vi "TANGO_Example_LV2011.vi"() -> ()   [LabVIEW 2018, in "TangoOWN.lvlib"]
uses:
  SubVIs/AxisControl.ctl
  SubVIs/Axis_Switch.ctl
  TangoOWN.lvlib
  SDK/Tango.lvlib
panel:
  out "CloseWindow":bool
  out "Limit Switches":T1[](array[typedef])
  in  "Calibrate":bool
  in  "RMeasure":bool
  in  "Center":bool
  in  "Tab_Control":enum32{"Control", "Low level"}(tab)
  in  "Analog Output2":i32(slide) scale=0.0..100.0
  in  "Analog Output1":i32(slide) scale=0.0..100.0
  in  "Move absolute":bool
  in  "Destination [mm]":dbl[](array[numeric]) format="%_6g"
  in  "Manual Control":T2[](array[typedef])
  in  "Step Width [mm]":dbl=1.0 min=0.0 format="%_6f"
  in  "Send":bool
  in  "Limits":bool
  out "Return Message":string
  in  "Command":string caption="Send Command"
  in  "Sequence":bool
  in  "Maeander":bool
  in  "Set Zero":bool
  in  "Velocity":bool
  out "MinRange":dbl[](array[numeric])
  out "MaxRange":dbl[](array[numeric])
  out "RMResult":dbl[](array[numeric])
  out "Position":dbl[](array[numeric]) format="%_6f"
  out "Number of Axis":u8=3
  in  "ShProt?":bool=TRUE caption="Show Protocol?"
  in  "Disconnect":bool
  out "Connected?":bool
  in  "Connect":bool
  in  "Baudrate":i32=57600
  in  "VISA-Ressourcename":refnum<visa-resource-name>
  out "Func-Return":i32
  in  "Stopp":bool
  out "error out":errorcluster
  out "State":string="Idle"
  in  "Fehler (Eingang, kein Fehler)":errorcluster
  # "TANGO Example v0.1"
  # "E0"
  # "EE"
  # "X"
  # "Y"
  # "Z"
  # "A"
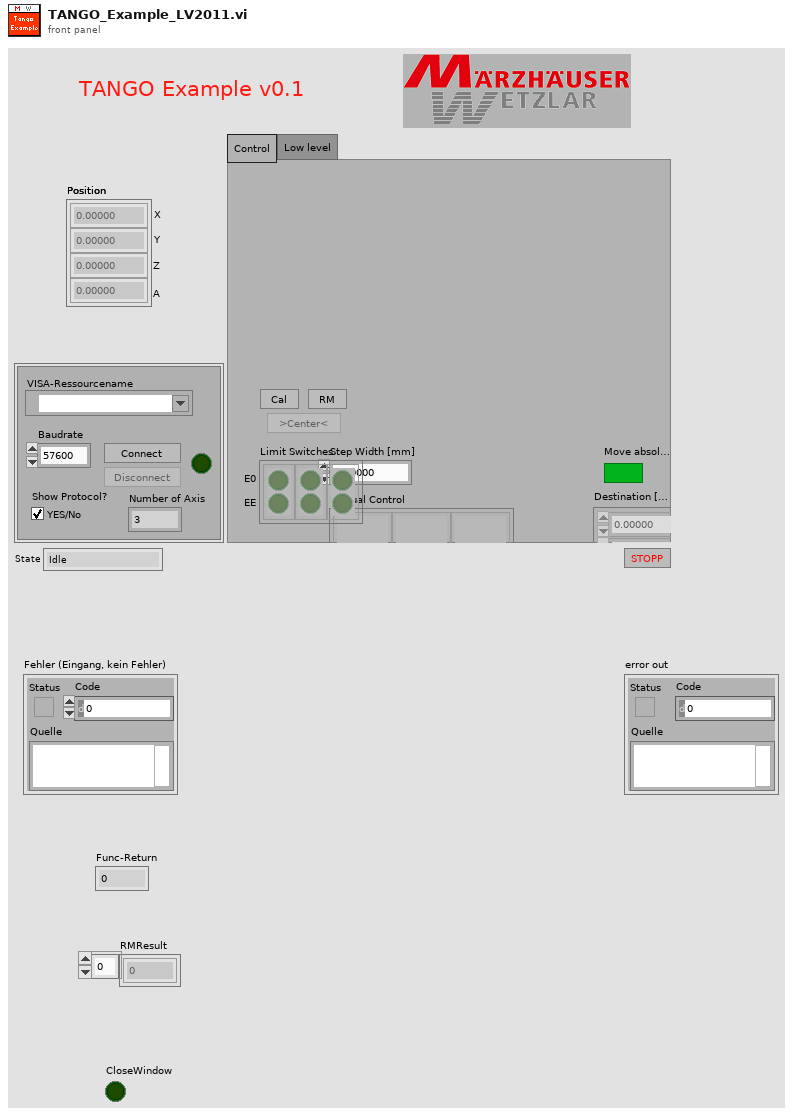
[diagram p1: front panel]
types:
  T1 = typedef "TangoOWN.lvlib/Axis_Switch.ctl" = cluster{"E0":bool, "EE":bool}
  T2 = typedef "TangoOWN.lvlib/AxisControl.ctl" = cluster{"Plus":bool, "Minus":bool}
  T3 = enum8{"Enabled", "Disabled", "Disabled and Grayed Out"}
  T4 = typedef "TangoOWN.lvlib/Maeander_Param.ctl" = cluster{"Number":i32, "X Start":dbl, "Y Start":dbl, "X Size":dbl, "Y Size":dbl}
  T5 = typedef "TangoOWN.lvlib/SequenceParam.ctl" = cluster{"Number of cycles":i32, "Start position":dbl[], "End position":dbl[]}
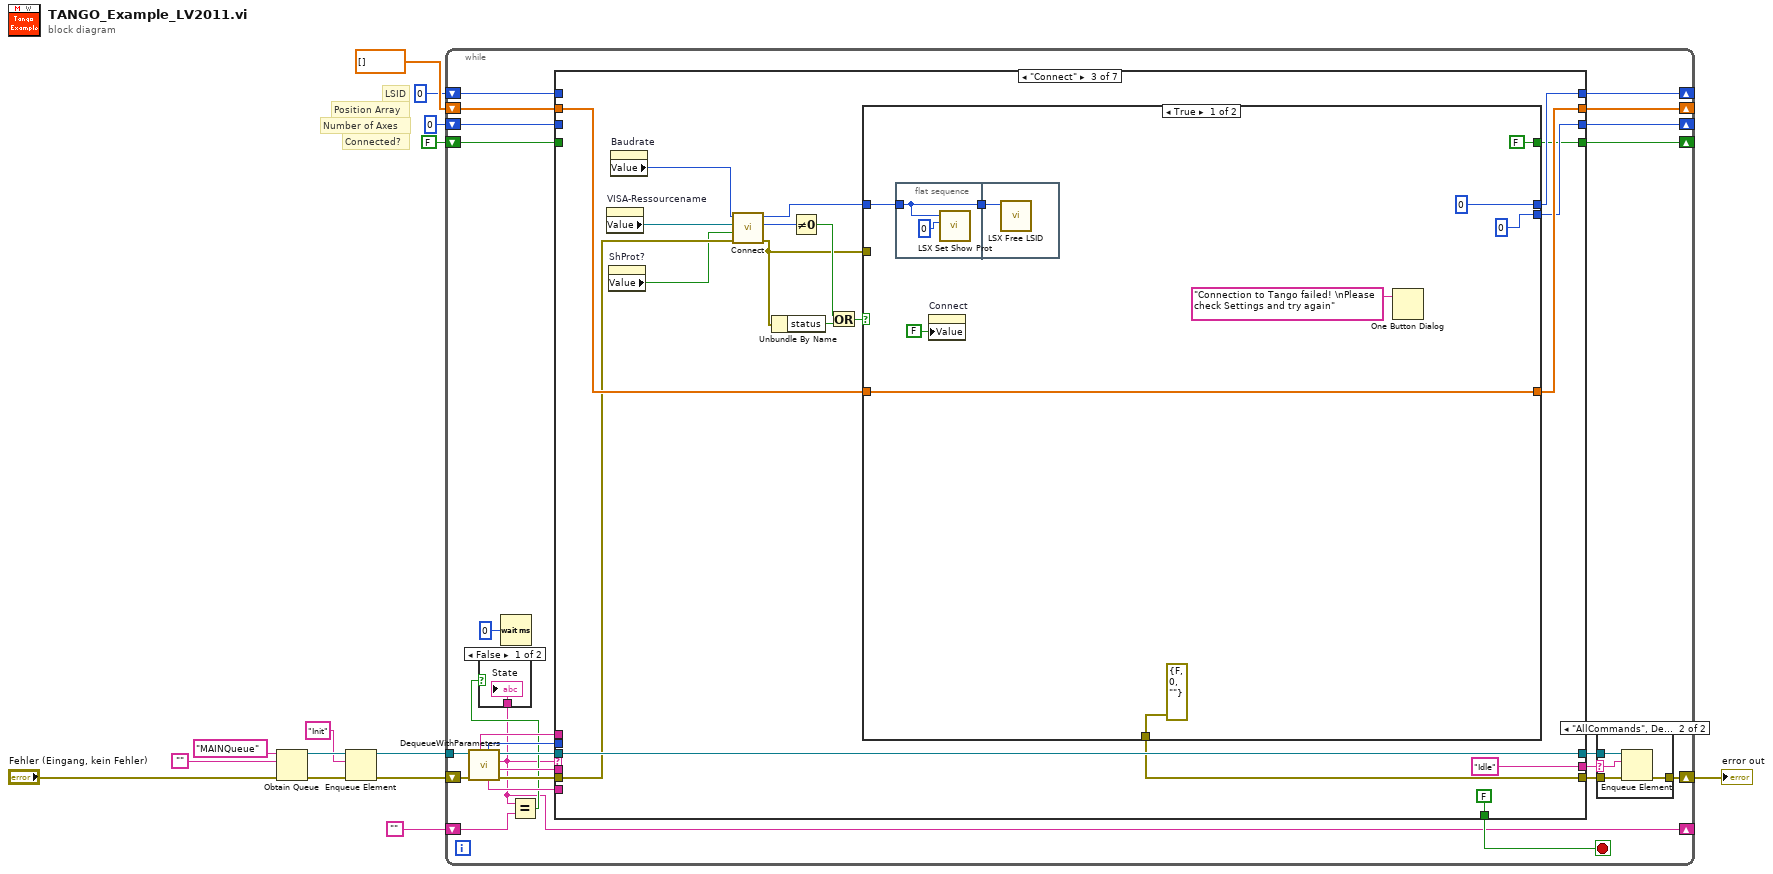
[diagram p0: block diagram]
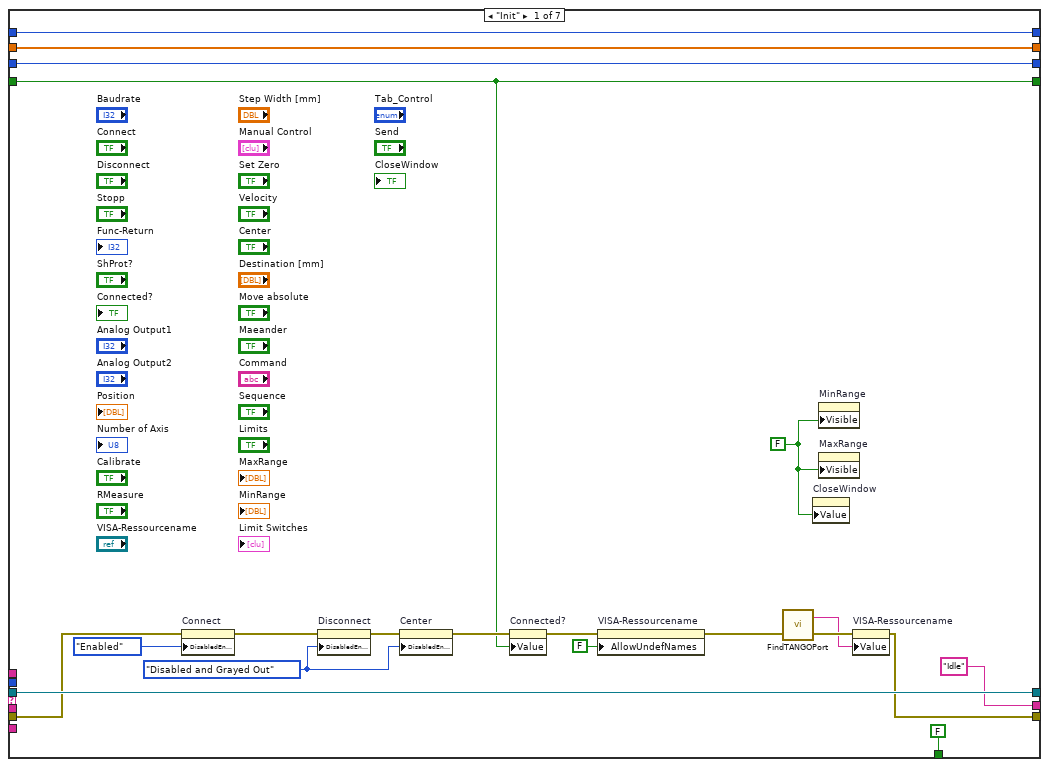
[diagram p4: hidden frame]
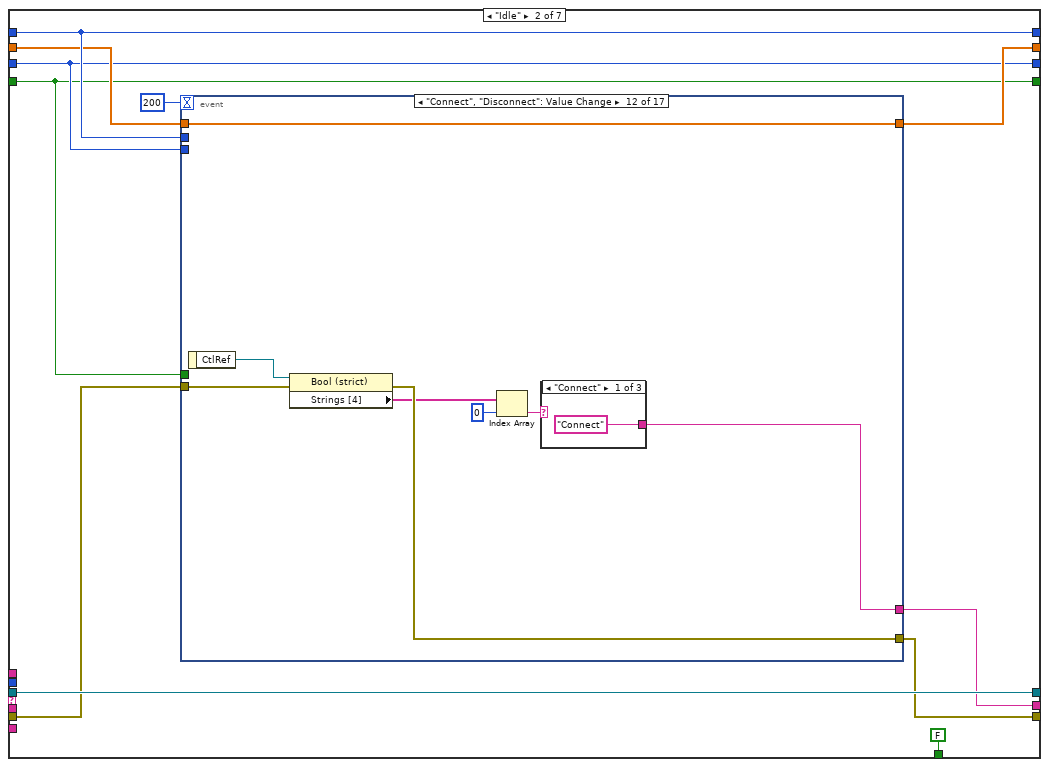
[diagram p5: hidden frame]
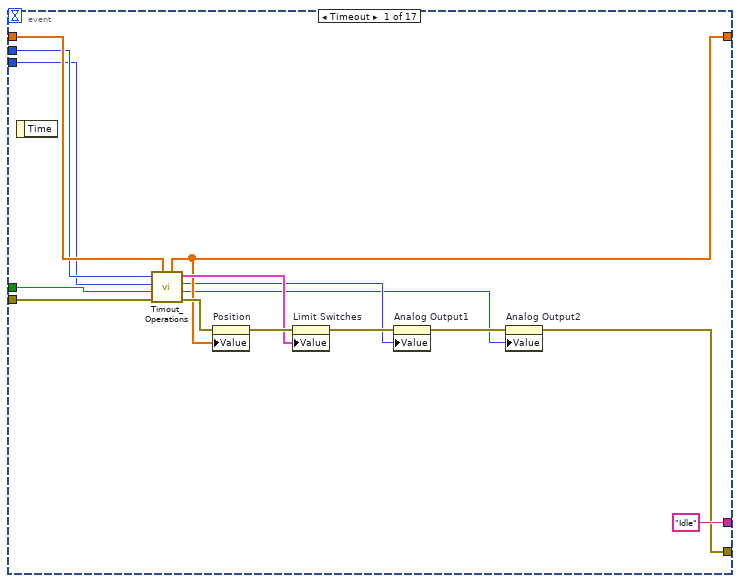
[diagram p6: hidden frame]
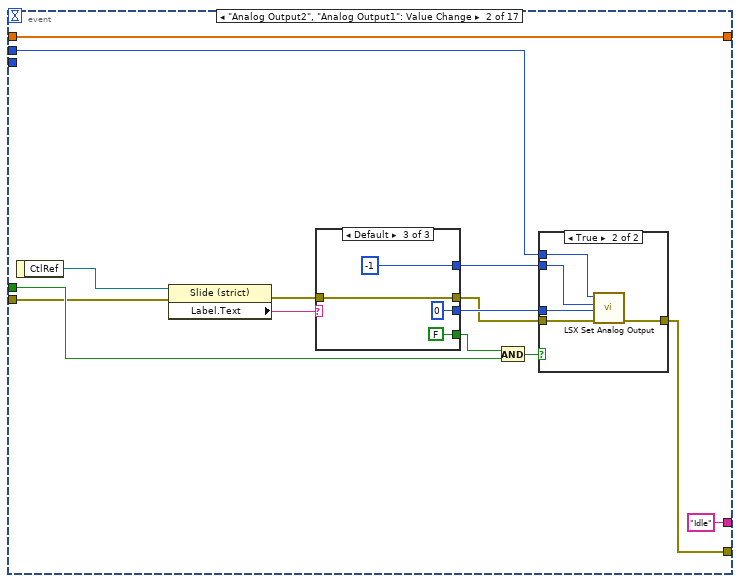
[diagram p7: hidden frame]
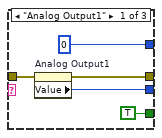
[diagram p8: hidden frame]
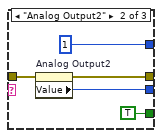
[diagram p9: hidden frame]
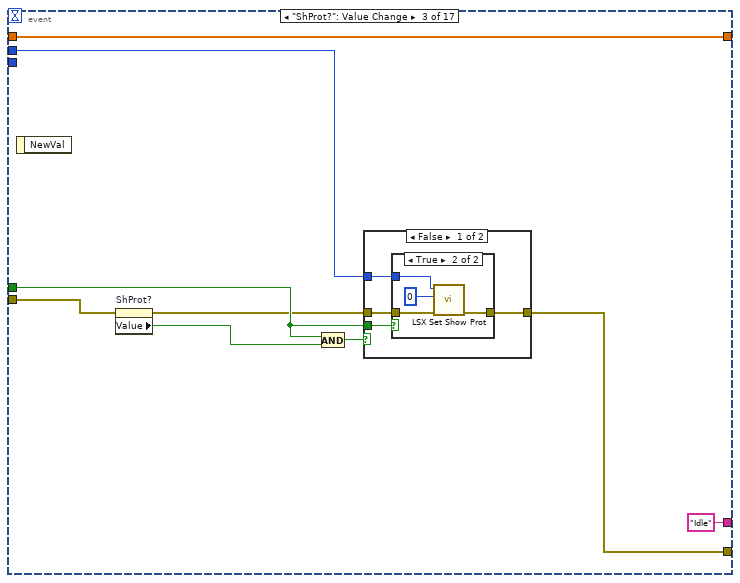
[diagram p11: hidden frame]
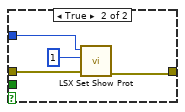
[diagram p13: hidden frame]
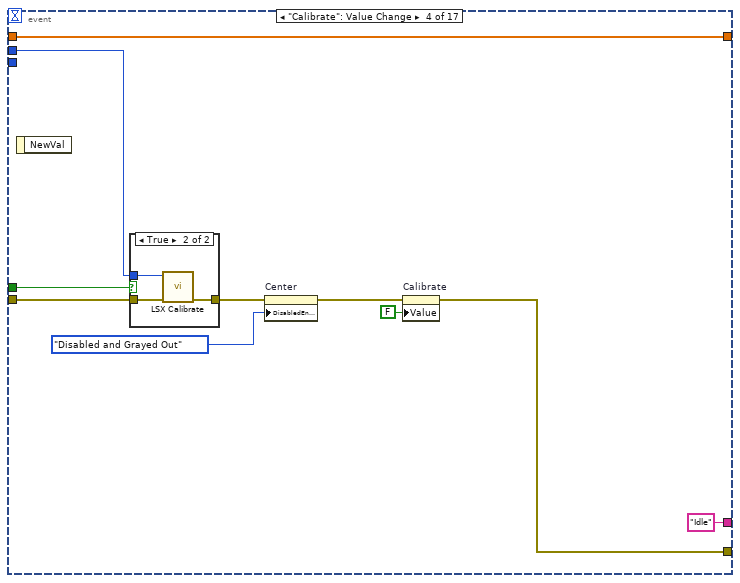
[diagram p14: hidden frame]
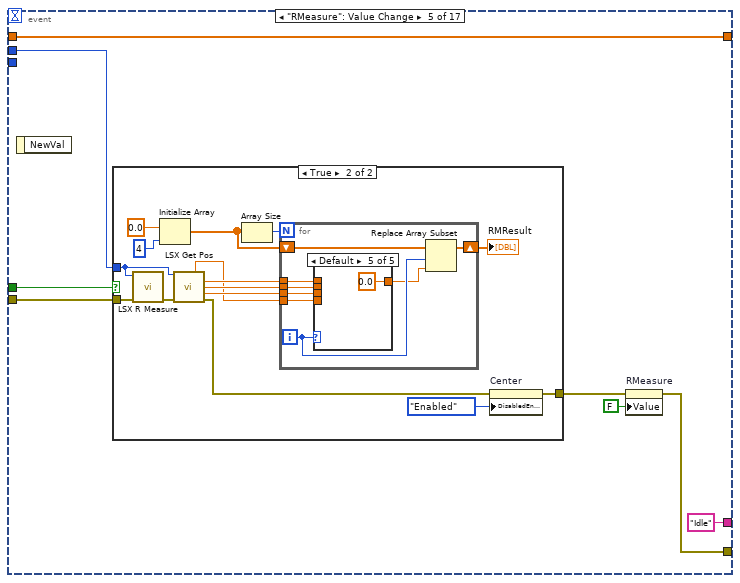
[diagram p16: hidden frame]
diagram:
  # "Connected?"
  # "Number of Axes"
  # "Position Array"
  # "LSID"
  n1 = Obtain Queue(name (unnamed)="MAINQueue" ("Name (unbenannt)"), element data type="", error in (no error)="Fehler (Eingang, kein Fehler)") -> (queue out=w11:refnum<queue>, error out=w10:errorcluster)  [unwired: 2 in, 1 out]
  n2 = Enqueue Element(queue=w11, element="Init" ("Element"), error in (no error)=w10) -> (queue out=w8:refnum<queue>, error out=w7:errorcluster)  [unwired: 1 in, 1 out]
  n3 = while {
    tunnel: w8 -> [w37]
    shift-right: [w24] -> w5
    shift-left: w7 -> [w38]
    shift-right: [w23] -> _
    shift-left: "" -> [w29]
    shift-right: [w22] -> _
    shift-left: 0 ("plLSID out") -> [w21]
    shift-right: [w20] -> _
    shift-left: dbl[] [] -> [w19]
    shift-right: [w17] -> _
    shift-left: u8 0 ("plLSID out") -> [w18]
    shift-right: [w15] -> _
    shift-left: FALSE -> [w16]
    stop <- w39 stop-if-true
    n4 = call "DequeueWithParameters.vi"("error in"=w38, "Queue in"=w37) -> ("error out"=w31:errorcluster, "channelStr"=w32:string, "command"=w23:string, "Queue out"=w35:refnum<queue>, "telegram"=w30:string, "channel"=w34:i32, "QueueCmd"=w33:string)  [unwired: 3 in]
    n5 = Wait (ms)(milliseconds to wait=u32 0) -> ()  [unwired: 1 out]
    n6 = Equal?(x=w23, y=w29) -> (x = y?=w28:bool)
    n7 = case shown="False" w28 {
      tunnel: w23 -> [w45 _]
      frame False {
        "State" <- w45
      }
      frame True {
      }
    }
    n8 = case shown="\"Connect\"" w23 {
      tunnel: [FALSE FALSE FALSE FALSE FALSE TRUE TRUE] -> w39
      tunnel: w35 -> [w64 w76 w529 w585 w597 w625 w654]
      tunnel: w34 -> [_ _ _ _ _ _ _]
      tunnel: w33 -> [_ _ _ _ _ _ _]
      tunnel: w32 -> [_ _ _ _ _ _ _]
      tunnel: w31 -> [w62 w67 w514 w581 w589 w609 w640]
      tunnel: w30 -> [_ _ _ _ _ _ _]
      tunnel: [w64 w76 w529 w585 w597 w625 refnum<queue> refnum ("Queue out")] -> w27
      tunnel: ["Idle" w73 "Idle" "Idle" "Idle" "" ""] -> w26
      tunnel: [w57 w74 w526 w572 w588 errorcluster {"status"=FALSE, "code"=0, "source"=""} ("error out") w636] -> w25
      tunnel: [w60 w71 w520 0 ("plLSID out") w593 0 ("plLSID out") 0 ("plLSID out")] -> w22
      tunnel: w21 -> [w60 w71 _ w582 w593 w620 w652]
      tunnel: [w59 w69 w525 w579 w596 w617 w645] -> w20
      tunnel: w19 -> [w59 w70 w524 w579 w596 w617 w645]
      tunnel: [w50 w68 w519 u8 0 ("plLSID out") w587 u8 0 ("plLSID out") u8 0 ("plLSID out")] -> w17
      tunnel: w18 -> [w50 w68 _ _ w587 _ _]
      tunnel: w16 -> [w47 w66 _ _ w586 w610 w641]
      tunnel: [w47 w66 w518 w569 w586 w611 w642] -> w15
      frame "Init" {
        w46 = FALSE
        w53 = T3."Disabled and Grayed Out" ("Deaktiviert")
        n9 = property on="Connect" class="Bool (strict)"(error in=w62, "DisabledEnum"=T3."Enabled" ("Deaktiviert")) -> (error out=w61:errorcluster)  [unwired: 1 in, 1 out]
        n10 = property on="Disconnect" class="Bool (strict)"(error in=w61, "DisabledEnum"=w53) -> (error out=w52:errorcluster)  [unwired: 1 in, 1 out]
        n11 = property on="Center" class="Bool (strict)"(error in=w52, "DisabledEnum"=w53) -> (error out=w49:errorcluster)  [unwired: 1 in, 1 out]
        n12 = property on="Connected?" class="Bool (strict)"(error in=w49, "Value"=w47) -> (error out=w48:errorcluster)  [unwired: 1 in, 1 out]
        n13 = property on="VISA-Ressourcename" class="VISAName"(error in=w48, "AllowUndefNames"=FALSE ("Undefinierte Namen möglich")) -> (error out=w51:errorcluster)  [unwired: 1 in, 1 out]
        n14 = call "FindTANGOPort.vi"("Fehler (Eingang, kein Fehler)"=w51) -> ("Fehler (Ausgang)"=w56:errorcluster, "TangoCOMPort"=w55:string)  [unwired: 1 in]
        n15 = property on="CloseWindow" class="Bool (strict)"("Value"=w46) -> ()  [unwired: 2 in, 2 out]
        n16 = property on="MinRange" class="Arr (strict)"("Visible"=w46) -> ()  [unwired: 2 in, 2 out]
        n17 = property on="MaxRange" class="Arr (strict)"("Visible"=w46) -> ()  [unwired: 2 in, 2 out]
        n18 = property on="VISA-Ressourcename" class="VISAName"(error in=w56, "Value"=w55) -> (error out=w57:errorcluster)  [unwired: 1 in, 1 out]
      }
      frame "Idle" {
        n19 = event shown="[11] \"Connect\", \"Disconnect\": Value Change" {
          selector: _ -> [_ _ _ _ _ _ _ _ _ _ _ _ _ _ _ _ _]
          dyn-events: _ -> [_ _ _ _ _ _ _ _ _ _ _ _ _ _ _ _ _]
          timeout: 200 -> [_ _ _ _ _ _ _ _ _ _ _ _ _ _ _ _ _]
          tunnel: [w77 w104 w131 w154 w165 w200 w286 w335 w359 w381 w401 w418 w424 w448 w467 w491 w494] -> w74
          tunnel: ["Idle" "Idle" "Idle" "Idle" "Idle" "Idle" "Idle" "Idle" "Idle" "Idle" "Idle" w414 w429 "Idle" "Idle" "Stop" w497] -> w73
          tunnel: w71 -> [w87 w105 w132 w155 w167 w202 w287 w338 w361 w382 w404 _ _ w445 w469 _ _]
          tunnel: w70 -> [w88 w103 w129 w157 w169 w206 w290 w342 w364 w384 w407 w413 w431 w451 w473 w492 w502]
          tunnel: [w82 w103 w129 w157 w169 w206 w290 w342 w364 w384 w407 w413 w431 w451 w473 w492 w502] -> w69
          tunnel: w66 -> [w89 w93 w128 w152 w163 w204 w285 w339 w363 w380 w406 _ w430 w447 w471 _ _]
          tunnel: w67 -> [w90 w92 w127 w151 w162 w203 w284 w340 w362 w379 w405 w412 w427 w446 w470 w491 w495]
          tunnel: w68 -> [w86 _ _ _ _ _ w283 _ _ _ _ _ _ w443 w465 _ _]
          event Timeout {
            n20 = event-data() -> ()  [unwired: 1 in, 1 out]
            n21 = call "Timout_Operations.vi"("PosIn"=w88, "error in"=w90, "Connected?"=w89, "NumberOfAxes"=w86, "plLSID"=w87) -> ("error out"=w85:errorcluster, "AnaOut2"=w78:i32, "Anaout1"=w79:i32, "LimitsOutput"=w83:T1[], "PosOut"=w82:dbl[])  [unwired: 2 in]
            n22 = property on="Position" class="Arr (strict)"(error in=w85, "Value"=w82) -> (error out=w84:errorcluster)  [unwired: 1 in, 1 out]
            n23 = property on="Limit Switches" class="Arr (strict)"(error in=w84, "Value"=w83) -> (error out=w81:errorcluster)  [unwired: 1 in, 1 out]
            n24 = property on="Analog Output1" class="Slide (strict)"(error in=w81, "Value"=w79) -> (error out=w80:errorcluster)  [unwired: 1 in, 1 out]
            n25 = property on="Analog Output2" class="Slide (strict)"(error in=w80, "Value"=w78) -> (error out=w77:errorcluster)  [unwired: 1 in, 1 out]
          }
          event "Analog Output2", "Analog Output1": Value Change {
            n26 = event-data() -> ("CtlRef"=w102:refnum<vi>)  [unwired: 1 in]
            n27 = property class="Slide (strict)"(reference=w102, error in=w92) -> (error out=w97:errorcluster, "Label.Text"=w101:string)  [unwired: 1 out]
            n28 = case shown="Default" w101 {
              tunnel: [0 1 -1] -> w98
              tunnel: [TRUE TRUE FALSE] -> w99
              tunnel: w97 -> [w108 w113 w117]
              tunnel: [w107 w112 w117] -> w95
              tunnel: [w106 w111 0 ("Value")] -> w96
              frame "Analog Output1" {
                n29 = property on="Analog Output1" class="Slide (strict)"(error in=w108) -> (error out=w107:errorcluster, "Value"=w106:i32)  [unwired: 1 in, 1 out]
              }
              frame "Analog Output2" {
                n30 = property on="Analog Output2" class="Slide (strict)"(error in=w113) -> (error out=w112:errorcluster, "Value"=w111:i32)  [unwired: 1 in, 1 out]
              }
              frame Default {
              }
            }
            n31 = And(x=w99, y=w93) -> (x .and. y?=w100:bool)
            n32 = case shown="True" w100 {
              tunnel: w105 -> [_ w125]
              tunnel: w95 -> [w120 w122]
              tunnel: [w120 w124] -> w104
              tunnel: w98 -> [_ w123]
              tunnel: w96 -> [_ w121]
              frame False {
              }
              frame True {
                n33 = call "LSX Set Analog Output.vi"("error in (no error)"=w122, "lValue"=w121, "lIndex"=w123, "lLSID"=w125) -> ("error out"=w124:errorcluster)  [unwired: 6 in, 1 out]
              }
            }
          }
          event "ShProt?": Value Change {
            n34 = event-data() -> ()  [unwired: 1 in, 1 out]
            n35 = property on="ShProt?" class="Bool (strict)"(error in=w127) -> (error out=w126:errorcluster, "Value"=w133:bool)  [unwired: 1 in, 1 out]
            n36 = And(x=w128, y=w133) -> (x .and. y?=w134:bool)
            n37 = case shown="False" w134 {
              tunnel: w126 -> [w137 w147]
              tunnel: w132 -> [w136 w145]
              tunnel: w128 -> [w138 _]
              tunnel: [w135 w144] -> w131
              frame False {
                n38 = case shown="True" w138 {
                  tunnel: w137 -> [w139 w143]
                  tunnel: w136 -> [_ w142]
                  tunnel: [w139 w140] -> w135
                  frame False {
                  }
                  frame True {
                    n39 = call "LSX Set Show Prot.vi"("error in (no error)"=w143, "bShowProt"=0, "lLSID"=w142) -> ("error out"=w140:errorcluster)  [unwired: 7 in, 1 out]
                  }
                }
              }
              frame True {
                n40 = call "LSX Set Show Prot.vi"("error in (no error)"=w147, "bShowProt"=1, "lLSID"=w145) -> ("error out"=w144:errorcluster)  [unwired: 7 in, 1 out]
              }
            }
          }
          event "Calibrate": Value Change {
            n41 = event-data() -> ()  [unwired: 1 in, 1 out]
            n42 = case shown="True" w152 {
              tunnel: w155 -> [_ w161]
              tunnel: [w158 w160] -> w150
              tunnel: w151 -> [w158 w159]
              frame False {
              }
              frame True {
                n43 = call "LSX Calibrate.vi"("error in (no error)"=w159, "lLSID"=w161) -> ("error out"=w160:errorcluster)  [unwired: 8 in, 1 out]
              }
            }
            n44 = property on="Center" class="Bool (strict)"(error in=w150, "DisabledEnum"=T3."Disabled and Grayed Out" ("Deaktiviert")) -> (error out=w148:errorcluster)  [unwired: 1 in, 1 out]
            n45 = property on="Calibrate" class="Bool (strict)"(error in=w148, "Value"=FALSE ("Calibrate")) -> (error out=w154:errorcluster)  [unwired: 1 in, 1 out]
          }
          event "RMeasure": Value Change {
            n46 = event-data() -> ()  [unwired: 1 in, 1 out]
            n47 = case shown="True" w163 {
              tunnel: w167 -> [_ w173]
              tunnel: [w170 w176] -> w166
              tunnel: w162 -> [w170 w172]
              frame False {
              }
              frame True {
                n48 = call "LSX R Measure.vi"("error in (no error)"=w172, "lLSID"=w173) -> ("error out"=w171:errorcluster)  [unwired: 8 in, 1 out]
                n49 = Initialize Array(0.0, 4 ("Dimension")) -> (w182:dbl[])
                n50 = call "LSX Get Pos.vi"("lLSID"=w173, "error in (no error)"=w171) -> ("pdA out"=w178:dbl, "pdX out"=w181:dbl, "pdY out"=w180:dbl, "pdZ out"=w179:dbl, "error out"=w175:errorcluster)  [unwired: 8 in, 1 out]
                n51 = Array Size(array=w182) -> (size(s)=w183:i32)
                n52 = for {
                  N: w183 -> [_]
                  tunnel: w181 -> [w192]
                  tunnel: w180 -> [w191]
                  tunnel: w179 -> [w190]
                  tunnel: w178 -> [w189]
                  shift-right: [w186] -> w177
                  shift-left: w182 -> [w193]
                  i -> [w188]
                  n53 = case shown="Default" w188 {
                    tunnel: w192 -> [w194 _ _ _ _]
                    tunnel: w191 -> [_ w195 _ _ _]
                    tunnel: w190 -> [_ _ w196 _ _]
                    tunnel: w189 -> [_ _ _ w197 _]
                    tunnel: [w194 w195 w196 w197 0.0 ("pdA out")] -> w187
                    frame 0 {
                    }
                    frame 1 {
                    }
                    frame 2 {
                    }
                    frame 3 {
                    }
                    frame Default {
                    }
                  }
                  n54 = Replace Array Subset(array=w193, new element=w187, index=w188) -> (w186:dbl[])
                }
                "RMResult" <- w177
                n55 = property on="Center" class="Bool (strict)"(error in=w175, "DisabledEnum"=T3."Enabled" ("Deaktiviert")) -> (error out=w176:errorcluster)  [unwired: 1 in, 1 out]
              }
            }
            n56 = property on="RMeasure" class="Bool (strict)"(error in=w166, "Value"=FALSE ("RMeasure")) -> (error out=w165:errorcluster)  [unwired: 1 in, 1 out]
          }
          event "Center": Value Change {
            n57 = event-data() -> ()  [unwired: 1 in, 1 out]
            n58 = case shown="True" w204 {
              tunnel: w203 -> [w207 w222]
              tunnel: w202 -> [_ w211]
              tunnel: [w207 w208] -> w201
              frame False {
              }
              frame True {
                w217 = 4
                w223 = 2
                w232 = 0 ("Index")
                n59 = call "LSX Get Switch Active.vi"("lLSID"=w211, "error in (no error)"=w222) -> ("plRA out"=w218:i32, "plXA out"=w221:i32, "plYA out"=w220:i32, "plZA out"=w219:i32, "error out"=w210:errorcluster)  [unwired: 8 in, 1 out]
                n60 = property on="RMResult" class="Arr (strict)"(error in=w210) -> (error out=w209:errorcluster, "Value"=w230:dbl[])  [unwired: 1 in, 1 out]
                n61 = Increment(x=w232) -> (x+1=w231:i32)
                n62 = for {
                  N: w217 -> [_]
                  tunnel: w221 -> [w264]
                  tunnel: w220 -> [w263]
                  tunnel: w219 -> [w262]
                  tunnel: w218 -> [w261]
                  tunnel: [w260] -> w216 mode=indexing
                  i -> [w265]
                  n63 = case shown="0" w265 {
                    tunnel: w264 -> [w267 _ _ _ _]
                    tunnel: w263 -> [_ w270 _ _ _]
                    tunnel: w262 -> [_ _ w274 _ _]
                    tunnel: w261 -> [_ _ _ w278 _]
                    tunnel: [w266 w271 w275 w279 FALSE] -> w260
                    frame 0 {
                      n64 = case shown="Default" w267 {
                        tunnel: [FALSE TRUE] -> w266
                        frame 0 {
                        }
                        frame Default {
                        }
                      }
                    }
                    frame 1 {
                      n65 = case shown="Default" w270 {
                        tunnel: [FALSE TRUE] -> w271
                        frame 0 {
                        }
                        frame Default {
                        }
                      }
                    }
                    frame 2 {
                      n66 = case shown="Default" w274 {
                        tunnel: [FALSE TRUE] -> w275
                        frame 0 {
                        }
                        frame Default {
                        }
                      }
                    }
                    frame 3 {
                      n67 = case shown="Default" w278 {
                        tunnel: [FALSE TRUE] -> w279
                        frame 0 {
                        }
                        frame Default {
                        }
                      }
                    }
                    frame Default {
                    }
                  }
                }
                n68 = Increment(x=w231) -> (x+1=w228:i32)
                n69 = Index Array(array=w230, index=w232) -> (element=w227:dbl)
                n70 = Index Array(array=w230, index=w231) -> (element=w226:dbl)
                n71 = Increment(x=w228) -> (x+1=w229:i32)
                n72 = Index Array(array=w230, index=w228) -> (element=w225:dbl)
                n73 = Index Array(array=w230, index=w229) -> (element=w224:dbl)
                n74 = Divide(x=w227, y=w223) -> (x/y=w215:dbl)
                n75 = Divide(x=w226, y=w223) -> (x/y=w214:dbl)
                n76 = Divide(x=w225, y=w223) -> (x/y=w213:dbl)
                n77 = Divide(x=w224, y=w223) -> (x/y=w212:dbl)
                n78 = for {
                  N: w217 -> [_]
                  tunnel: w216 -> [w242]
                  tunnel: w215 -> [w237]
                  tunnel: w214 -> [w236]
                  tunnel: w213 -> [w235]
                  tunnel: w212 -> [w234]
                  tunnel: w211 -> [w240]
                  tunnel: w209 -> [w239]
                  tunnel: [w233] -> w208
                  i -> [w238]
                  n79 = Index Array(array=w242, index=w238) -> (element=w241:bool)
                  n80 = case shown="True" w241 {
                    tunnel: w238 -> [_ w254]
                    tunnel: w240 -> [_ w252]
                    tunnel: w239 -> [w243 w251]
                    tunnel: w238 -> [_ w250]
                    tunnel: w237 -> [_ w249]
                    tunnel: w236 -> [_ w248]
                    tunnel: w235 -> [_ w247]
                    tunnel: w234 -> [_ w246]
                    tunnel: [w243 w244] -> w233
                    frame False {
                    }
                    frame True {
                      n81 = Increment(x=w254) -> (x+1=w253:i32)
                      n82 = case shown="Default" w250 {
                        tunnel: w249 -> [w255 _ _ _ _]
                        tunnel: w248 -> [_ w256 _ _ _]
                        tunnel: w247 -> [_ _ w257 _ _]
                        tunnel: w246 -> [_ _ _ w258 _]
                        tunnel: [w255 w256 w257 w258 0.0] -> w245
                        frame 0 {
                        }
                        frame 1 {
                        }
                        frame 2 {
                        }
                        frame 3 {
                        }
                        frame Default {
                        }
                      }
                      n83 = call "LSX Move Abs Single Axis.vi"("error in (no error)"=w251, "dValue"=w245, "lAxis"=w253, "lLSID"=w252) -> ("error out"=w244:errorcluster)  [unwired: 6 in, 1 out]
                    }
                  }
                }
              }
            }
            n84 = property on="Center" class="Bool (strict)"(error in=w201, "Value"=FALSE ("Center")) -> (error out=w200:errorcluster)  [unwired: 1 in, 1 out]
          }
          event "Manual Control": Value Change {
            n85 = event-data() -> ("CtlRef"=w288:refnum<vi>)  [unwired: 1 in]
            n86 = case shown="True" w285 {
              tunnel: w288 -> [_ w297]
              tunnel: w287 -> [_ w302]
              tunnel: [w291 w293] -> w286
              tunnel: w284 -> [w291 w298]
              tunnel: w283 -> [_ w292]
              frame False {
              }
              frame True {
                n87 = property class="Arr"(reference=w297, error in=w298) -> (error out=w299:errorcluster, "Value"=w313:variant)  [unwired: 1 out]
                n88 = Variant To Data(type=T2[] [], Variant=w313) -> (data=w296:T2[])  [unwired: 1 in, 1 out]
                n89 = for {
                  N: w292 -> [_]
                  tunnel: w296 -> [w317] mode=indexing
                  shift-right: [w319] -> w310
                  shift-left: -1 -> [w320]
                  shift-right: [w318] -> w308
                  shift-left: FALSE ("Minus") -> [_]
                  shift-right: [w314] -> w295
                  shift-left: w296 -> [w315]
                  i -> [w321]
                  stop <- w316 stop-if-true
                  n90 = stacked-sequence {
                    tunnel: w321 -> [w328 w331]
                    tunnel: w320 -> [w327 _]
                    tunnel: [w326 _] -> w319
                    tunnel: [w322 _] -> _
                    tunnel: [w325 _] -> w318
                    tunnel: w317 -> [w324 w334]
                    tunnel: [w322 _] -> w316
                    tunnel: w315 -> [_ w332]
                    tunnel: [_ w329] -> w314
                    frame #0 {
                      n91 = Unbundle By Name(w324) -> ("Plus"=w323:bool, "Minus"=w325:bool)
                      n92 = Or(x=w323, y=w325) -> (x .or. y?=w322:bool)
                      n93 = Select(t=w328, s=w322, f=w327) -> (s? t:f=w326:i32)
                    }
                    frame #1 {
                      w333 = FALSE
                      n94 = Bundle By Name(cluster=w334, "Plus"=w333, "Minus"=w333) -> (w330:T2)
                      n95 = Replace Array Subset(array=w332, new element=w330, index=w331) -> (w329:T2[])
                    }
                  }
                }
                n96 = property on="Step Width [mm]" class="DigNum (strict)"(error in=w299) -> (error out=w300:errorcluster, "Value"=w304:dbl)  [unwired: 1 in, 1 out]
                n97 = Increment(x=w310) -> (x+1=w303:i32)
                n98 = Select(t=-1, s=w308, f=1) -> (s? t:f=w305:i32)
                n99 = Multiply(x=w305, y=w304) -> (x*y=w301:dbl)
                n100 = call "LSX Move Rel Single Axis.vi"("error in (no error)"=w300, "dValue"=w301, "lAxis"=w303, "lLSID"=w302) -> ("error out"=w294:errorcluster)  [unwired: 6 in, 1 out]
                n101 = property class="Arr"(reference=w297, error in=w294, "Value"=w295) -> (error out=w293:errorcluster)  [unwired: 1 out]
              }
            }
          }
          event "Move absolute": Value Change {
            n102 = event-data() -> ()  [unwired: 1 in, 1 out]
            n103 = case shown="True" w339 {
              tunnel: w340 -> [w343 w356]
              tunnel: w338 -> [_ w349]
              tunnel: [w343 w344] -> w337
              frame False {
              }
              frame True {
                w353 = 0
                n104 = property on="Destination [mm]" class="Arr (strict)"(error in=w356) -> (error out=w350:errorcluster, "Value"=w355:dbl[])  [unwired: 1 in, 1 out]
                n105 = Increment(x=w353) -> (x+1=w352:i32)
                n106 = Increment(x=w352) -> (x+1=w351:i32)
                n107 = Increment(x=w351) -> (x+1=w354:i32)
                n108 = Index Array(array=w355, index=w353) -> (element=w348:dbl)
                n109 = Index Array(array=w355, index=w352) -> (element=w347:dbl)
                n110 = Index Array(array=w355, index=w351) -> (element=w346:dbl)
                n111 = Index Array(array=w355, index=w354) -> (element=w345:dbl)
                n112 = call "LSX Move Abs.vi"("dA"=w345, "dZ"=w346, "error in (no error)"=w350, "dY"=w347, "dX"=w348, "lLSID"=w349) -> ("error out"=w344:errorcluster)  [unwired: 4 in, 1 out]
              }
            }
            n113 = property on="Move absolute" class="Bool (strict)"(error in=w337, "Value"=FALSE ("Move absolute")) -> (error out=w335:errorcluster)  [unwired: 1 in, 1 out]
          }
          event "Maeander": Value Change {
            n114 = event-data() -> ()  [unwired: 1 in, 1 out]
            n115 = case shown="True" w363 {
              tunnel: w362 -> [w365 w371]
              tunnel: w361 -> [_ w369]
              tunnel: [w365 w366] -> w358
              frame False {
              }
              frame True {
                n116 = call "MaeanderDemo_Dlg.vi"("error in (no error)"=w371) -> ("error out"=w367:errorcluster, "Maeander Parameter"=w368:T4, "OK Out"=w370:bool)  [unwired: 8 in]
                n117 = case shown="True" w370 {
                  tunnel: w369 -> [_ w376]
                  tunnel: w368 -> [_ w375]
                  tunnel: w367 -> [w372 w374]
                  tunnel: [w372 w373] -> w366
                  frame False {
                  }
                  frame True {
                    n118 = call "MaeanderDemo.vi"("lLSID"=w376, "Maeander Parameter"=w375, "error in (no error)"=w374) -> ("error out"=w373:errorcluster)  [unwired: 6 in]
                  }
                }
              }
            }
            n119 = property on="Maeander" class="Bool (strict)"(error in=w358, "Value"=FALSE ("Mäander")) -> (error out=w359:errorcluster)  [unwired: 1 in, 1 out]
          }
          event "Set Zero": Value Change {
            n120 = event-data() -> ()  [unwired: 1 in, 1 out]
            n121 = case shown="True" w380 {
              tunnel: w382 -> [_ w392]
              tunnel: w379 -> [w385 w391]
              tunnel: [w385 w386] -> w377
              frame False {
              }
              frame True {
                n122 = Two Button Dialog(message="Are you sure?" ("Nachricht"), 1:"No" ("Text für F-Schaltfläche (\"Abbrechen\")"), 2:"Yes" ("Text für T-Schaltfläche (\"OK\")")) -> (T button?=w387:bool)
                n123 = case shown="True" w387 {
                  tunnel: w392 -> [_ w395]
                  tunnel: w391 -> [w393 w397]
                  tunnel: [w393 w399] -> w386
                  frame False {
                  }
                  frame True {
                    w394 = 0.0 ("dX")
                    n124 = call "LSX Set Pos.vi"("dA"=w394, "dZ"=w394, "error in (no error)"=w397, "dY"=w394, "dX"=w394, "lLSID"=w395) -> ("error out"=w396:errorcluster)  [unwired: 4 in, 1 out]
                    n125 = property on="Center" class="Bool (strict)"(error in=w396, "DisabledEnum"=T3."Disabled and Grayed Out" ("Deaktiviert")) -> (error out=w399:errorcluster)  [unwired: 1 in, 1 out]
                  }
                }
              }
            }
            n126 = property on="Set Zero" class="Bool (strict)"(error in=w377, "Value"=FALSE ("Set Zero")) -> (error out=w381:errorcluster)  [unwired: 1 in, 1 out]
          }
          event "Velocity": Value Change {
            n127 = event-data() -> ()  [unwired: 1 in, 1 out]
            n128 = case shown="True" w406 {
              tunnel: w405 -> [w408 w411]
              tunnel: w404 -> [_ w410]
              tunnel: [w408 w409] -> w402
              frame False {
              }
              frame True {
                n129 = call "DialogSpeed.vi"("error in (no error)"=w411, "lLSID"=w410) -> ("error out"=w409:errorcluster)
              }
            }
            n130 = property on="Velocity" class="Bool (strict)"(error in=w402, "Value"=FALSE ("Velocity")) -> (error out=w401:errorcluster)  [unwired: 1 in, 1 out]
          }
          event "Connect", "Disconnect": Value Change {
            n131 = event-data() -> ("CtlRef"=w419:refnum<vi>)  [unwired: 1 in]
            n132 = property class="Bool (strict)"(reference=w419, error in=w412) -> (error out=w418:errorcluster, "Strings [4]"=w417:string[])  [unwired: 1 out]
            n133 = Index Array(array=w417, index=0 ("Index")) -> (element=w416:string)
            n134 = case shown="\"Connect\"" w416 {
              tunnel: ["Connect" "Disconnect" "Idle"] -> w414
              frame "Connect" {
              }
              frame "Disconnect" {
              }
              frame Default {
              }
            }
          }
          event "Send": Value Change {
            n135 = event-data() -> ()  [unwired: 1 in, 1 out]
            n136 = property on="Command" class="Str"(error in=w427) -> (error out=w426:errorcluster, "Value"=w428:string)  [unwired: 1 in, 1 out]
            n137 = case shown="True" w430 {
              tunnel: w426 -> [w433 w438]
              tunnel: ["Idle" w435] -> w429
              tunnel: [w433 w434] -> w425
              tunnel: w428 -> [_ w437]
              frame False {
              }
              frame True {
                n138 = Empty String/Path?(string/path=w437) -> (empty?=w436:bool)
                n139 = case shown="False" w436 {
                  tunnel: ["SendCommand" "Idle"] -> w435
                  tunnel: w438 -> [w440 w441]
                  tunnel: [w440 w441] -> w434
                  frame False {
                  }
                  frame True {
                  }
                }
              }
            }
            n140 = property on="Send" class="Bool (strict)"(error in=w425, "Value"=FALSE ("Send")) -> (error out=w424:errorcluster)  [unwired: 1 in, 1 out]
          }
          event "Sequence": Value Change {
            n141 = event-data() -> ()  [unwired: 1 in, 1 out]
            n142 = case shown="True" w447 {
              tunnel: w446 -> [w452 w453]
              tunnel: w445 -> [_ w456]
              tunnel: [w452 w455] -> w444
              tunnel: w443 -> [_ w454]
              frame False {
              }
              frame True {
                n143 = call "SequenceDemo_dlg.vi"("error in (no error)"=w453, "NumberOfAxes"=w454) -> ("error out"=w457:errorcluster, "Sequence Paras"=w458:T5, "OK Out"=w459:bool)  [unwired: 7 in]
                n144 = case shown="True" w459 {
                  tunnel: w458 -> [_ w462]
                  tunnel: w457 -> [w460 w464]
                  tunnel: w456 -> [_ w463]
                  tunnel: [w460 w461] -> w455
                  frame False {
                  }
                  frame True {
                    n145 = call "SequenceDemo.vi"("error in (no error)"=w464, "Sequence Paras"=w462, "lLSID"=w463) -> ("error out"=w461:errorcluster)  [unwired: 8 in]
                  }
                }
              }
            }
            n146 = property on="Sequence" class="Bool (strict)"(error in=w444, "Value"=FALSE ("Sequence")) -> (error out=w448:errorcluster)  [unwired: 1 in, 1 out]
          }
          event "Limits": Value Change {
            n147 = event-data() -> ()  [unwired: 1 in, 1 out]
            n148 = case shown="True" w471 {
              tunnel: w470 -> [w474 w477]
              tunnel: w469 -> [_ w483]
              tunnel: [w474 w482] -> w468
              tunnel: w465 -> [_ w476]
              frame False {
              }
              frame True {
                w475 = TRUE
                n149 = property on="MinRange" class="Arr (strict)"("Number of Rows"=w476) -> ()  [unwired: 2 in, 2 out]
                n150 = property on="MaxRange" class="Arr (strict)"("Number of Rows"=w476) -> ()  [unwired: 2 in, 2 out]
                n151 = for {
                  N: w476 -> [_]
                  tunnel: w483 -> [w489]
                  shift-right: [w488] -> w480
                  shift-left: w477 -> [w490]
                  tunnel: [w485] -> w479 mode=indexing
                  tunnel: [w484] -> w478 mode=indexing
                  i -> [w486]
                  n152 = Increment(x=w486) -> (x+1=w487:i32)
                  n153 = call "LSX Get Limit.vi"("error in (no error)"=w490, "lAxis"=w487, "lLSID"=w489) -> ("error out"=w488:errorcluster, "pdMinRange out"=w485:dbl, "pdMaxRange out"=w484:dbl)  [unwired: 5 in, 1 out]
                }
                n154 = property on="MinRange" class="Arr (strict)"(error in=w480, "Value"=w479) -> (error out=w481:errorcluster)  [unwired: 1 in, 1 out]
                n155 = property on="MinRange" class="Arr (strict)"("Visible"=w475) -> ()  [unwired: 2 in, 2 out]
                n156 = property on="MaxRange" class="Arr (strict)"("Visible"=w475) -> ()  [unwired: 2 in, 2 out]
                n157 = property on="MaxRange" class="Arr (strict)"(error in=w481, "Value"=w478) -> (error out=w482:errorcluster)  [unwired: 1 in, 1 out]
              }
            }
            n158 = property on="Limits" class="Bool (strict)"(error in=w468, "Value"=FALSE ("Switches")) -> (error out=w467:errorcluster)  [unwired: 1 in, 1 out]
          }
          event "Stopp": Value Change {
            n159 = event-data() -> ()  [unwired: 1 in, 1 out]
          }
          event Panel Close? {
            n160 = event-data() -> ()  [unwired: 1 in, 1 out]
            n161 = Two Button Dialog(message="Are you sure you want to quit?" ("Nachricht"), 1:"No" ("Text für F-Schaltfläche (\"Abbrechen\")"), 2:"Yes" ("Text für T-Schaltfläche (\"OK\")")) -> (T button?=w498:bool)
            n162 = case shown="False" w498 {
              tunnel: ["Idle" "Stop"] -> w497
              tunnel: [w504 w508] -> w494
              tunnel: w495 -> [w503 w509]
              frame False {
                n163 = property on="CloseWindow" class="Bool (strict)"(error in=w503, "Value"=FALSE ("CloseWindow")) -> (error out=w504:errorcluster)  [unwired: 1 in, 1 out]
              }
              frame True {
                n164 = property on="CloseWindow" class="Bool (strict)"(error in=w509, "Value"=TRUE ("CloseWindow")) -> (error out=w508:errorcluster)  [unwired: 1 in, 1 out]
              }
            }
            n165 = event-data("Discard?"=TRUE ("Verwerfen?")) -> ()  [unwired: 1 in, 1 out]
          }
        }
      }
      frame "Connect" {
        n166 = property on="VISA-Ressourcename" class="VISAName"() -> ("Value"=w513:refnum<visa-resource-name>)  [unwired: 2 in, 2 out]
        n167 = property on="ShProt?" class="Bool (strict)"() -> ("Value"=w511:bool)  [unwired: 2 in, 2 out]
        n168 = property on="Baudrate" class="DigNum (strict)"() -> ("Value"=w515:i32)  [unwired: 2 in, 2 out]
        n169 = call "Connect.vi"("error in (no error)"=w514, "ShProt?"=w511, "pcAComName"=w513, "lABaudRate"=w515) -> ("error out"=w512:errorcluster, "function return"=w517:i32, "plLSID out"=w516:i32)  [unwired: 4 in]
        n170 = Unbundle By Name(w512) -> ("status"=w521:bool)
        n171 = Not Equal To 0?(x=w517) -> (x != 0?=w522:bool)
        n172 = Or(x=w522, y=w521) -> (x .or. y?=w523:bool)
        n173 = case shown="True" w523 {
          tunnel: [errorcluster {"status"=FALSE, "code"=0, "source"=""} ("Fehler (Ausgang)") w542] -> w526
          tunnel: [w537 w558] -> w525
          tunnel: w524 -> [w537 _]
          tunnel: w512 -> [_ w552]
          tunnel: w516 -> [w534 w543]
          tunnel: [0 ("plLSID out") w543] -> w520
          tunnel: [u8 0 w545] -> w519
          tunnel: [FALSE ("Connected?") w544] -> w518
          frame True {
            n174 = flat-sequence {
              tunnel: w534 -> [w539]
              tunnel: [w539] -> w535
              tunnel: w535 -> [w541]
              frame #0 {
                n175 = call "LSX Set Show Prot.vi"("bShowProt"=0, "lLSID"=w539) -> ()  [unwired: 8 in, 2 out]
              }
              frame #1 {
                n176 = call "LSX Free LSID.vi"("lLSID"=w541) -> ()  [unwired: 9 in, 2 out]
              }
            }
            n177 = property on="Connect" class="Bool (strict)"("Value"=FALSE ("Connect")) -> ()  [unwired: 2 in, 2 out]
            n178 = One Button Dialog(message="Connection to Tango failed! \nPlease check Settings and try again" ("Nachricht")) -> ()  [unwired: 1 in, 1 out]
          }
          frame False {
            w544 = TRUE ("Connected?")
            n179 = call "LSX Get Active Axes.vi"("error in (no error)"=w552, "lLSID"=w543) -> ("error out"=w548:errorcluster, "plFlags out"=w551:i32)  [unwired: 7 in, 1 out]
            n180 = Number To Boolean Array(number=w551) -> (Boolean array=w550:bool[])
            n181 = for {
              tunnel: w550 -> [w565] mode=indexing
              shift-right: [w563] -> w545
              shift-left: u8 0 -> [w564]
              tunnel: [w562] -> w542
              tunnel: w548 -> [w562]
              n182 = case shown="True" w565 {
                tunnel: w564 -> [w566 w568]
                tunnel: [w566 w567] -> w563
                frame False {
                }
                frame True {
                  n183 = Increment(x=w568) -> (x+1=w567:u8)
                }
              }
            }
            n184 = Initialize Array(0.0, w545) -> (w553:dbl[])
            n185 = Initialize Array(T2 {"Plus"=FALSE, "Minus"=FALSE} ("AxisControl"), w545) -> (w557:T2[])
            n186 = Initialize Array(T1 {"E0"=FALSE, "EE"=FALSE} ("Switch"), w545) -> (w546:T1[])
            n187 = property on="Destination [mm]" class="Arr (strict)"("Value"=w553) -> ()  [unwired: 2 in, 2 out]
            n188 = property on="Number of Axis" class="DigNum (strict)"("Value"=w545) -> ()  [unwired: 2 in, 2 out]
            n189 = property on="Destination [mm]" class="Arr (strict)"("Number of Rows"=w545) -> ()  [unwired: 2 in, 2 out]
            n190 = property on="Manual Control" class="Arr"("Number of Columns"=w545) -> ()  [unwired: 2 in, 2 out]
            n191 = property on="Manual Control" class="Arr"("Value"=w557) -> ()  [unwired: 2 in, 2 out]
            n192 = Initialize Array(0.0 ("Element"), w545) -> (w558:dbl[])
            n193 = property on="Connected?" class="Bool (strict)"("Value"=w544) -> ()  [unwired: 2 in, 2 out]
            n194 = property on="Connect" class="Bool (strict)"("DisabledEnum"=T3."Disabled and Grayed Out" ("Deaktiviert"), "Value"=FALSE ("Connect")) -> ()  [unwired: 2 in, 2 out]
            n195 = property on="Disconnect" class="Bool (strict)"("DisabledEnum"=T3."Enabled" ("Deaktiviert")) -> ()  [unwired: 2 in, 2 out]
            n196 = property on="Limit Switches" class="Arr (strict)"("Value"=w546, "Number of Columns"=w545) -> ()  [unwired: 2 in, 2 out]
          }
        }
      }
      frame "Disconnect" {
        w576 = T3."Disabled and Grayed Out" ("Deaktiviert")
        w569 = FALSE ("Connected?")
        n197 = call "Disconnect.vi"("error in (no error)"=w581, "lLSID"=w582) -> ("error out"=w580:errorcluster)
        n198 = property on="Connect" class="Bool (strict)"(error in=w580, "DisabledEnum"=T3."Enabled" ("Deaktiviert")) -> (error out=w571:errorcluster)  [unwired: 1 in, 1 out]
        n199 = property on="Connected?" class="Bool (strict)"(error in=w571, "Value"=w569) -> (error out=w570:errorcluster)  [unwired: 1 in, 1 out]
        n200 = property on="Disconnect" class="Bool (strict)"(error in=w570, "DisabledEnum"=w576, "Value"=FALSE ("Disconnect")) -> (error out=w577:errorcluster)  [unwired: 1 in, 1 out]
        n201 = property on="Center" class="Bool (strict)"(error in=w577, "DisabledEnum"=w576) -> (error out=w572:errorcluster)  [unwired: 1 in, 1 out]
      }
      frame "SendCommand" {
        n202 = property on="Command" class="Str"(error in=w589) -> (error out=w591:errorcluster, "Value"=w590:string)  [unwired: 1 in, 1 out]
        n203 = Empty String/Path?(string/path=w590) -> (empty?=w592:bool)
        n204 = case shown="True" w592 {
          tunnel: w593 -> [w607 _]
          tunnel: w591 -> [w605 w608]
          tunnel: w590 -> [w602 _]
          tunnel: [w598 w608] -> w588
          frame False {
            n205 = Concatenate Strings(w602, "\r") -> (w603:string)
            n206 = call "LSX Send String.vi"("lLSID"=w607, "bReadLine"=1, "pcStr"=w603, "lMaxLen"=256, "error in (no error)"=w605, "lTimeOut"=1000) -> ("pcRet out"=→"Return Message":string, "error out"=w598:errorcluster)  [unwired: 6 in, 2 out]
          }
          frame True {
          }
        }
      }
      frame "Error", Default {
        w616 = T3."Disabled and Grayed Out" ("Deaktiviert")
        w611 = FALSE ("Connected?")
        n207 = Unbundle By Name(w609) -> ("status"=w624:bool)
        n208 = case shown="True" w610 {
          tunnel: w620 -> [_ w627]
          tunnel: w609 -> [_ w626]
          frame False {
          }
          frame True {
            n209 = call "Disconnect.vi"("error in (no error)"=w626, "lLSID"=w627) -> ()  [unwired: 1 out]
          }
        }
        n210 = property on="Connect" class="Bool (strict)"(error in=w609, "DisabledEnum"=T3."Enabled" ("Deaktiviert")) -> (error out=w619:errorcluster)  [unwired: 1 in, 1 out]
        n211 = case shown="True" w624 {
          tunnel: w609 -> [_ w635]
          frame False {
          }
          frame True {
            n212 = Unbundle By Name(w635) -> ("code"=w634:i32, "source"=w633:string)  [unwired: 1 out]
            n213 = Number To Decimal String(number=w634) -> (decimal integer string=w631:string)  [unwired: 1 in]
            n214 = Concatenate Strings("Error!\n\nCode: ", w631, "\r\n", "Source: ", w633) -> (w628:string)
            n215 = One Button Dialog(message=w628) -> ()  [unwired: 1 in, 1 out]
          }
        }
        n216 = property on="Disconnect" class="Bool (strict)"(error in=w619, "DisabledEnum"=w616) -> (error out=w613:errorcluster)  [unwired: 1 in, 1 out]
        n217 = property on="Connected?" class="Bool (strict)"(error in=w613, "Value"=w611) -> (error out=w612:errorcluster)  [unwired: 1 in, 1 out]
        n218 = property on="Center" class="Bool (strict)"(error in=w612, "DisabledEnum"=w616) -> ()  [unwired: 1 in, 2 out]
      }
      frame "Stop" {
        w642 = FALSE ("Connected?")
        n219 = case shown="True" w641 {
          tunnel: w652 -> [_ w668]
          tunnel: w640 -> [w665 w667]
          tunnel: [w665 w666] -> w647
          frame False {
          }
          frame True {
            n220 = call "Disconnect.vi"("error in (no error)"=w667, "lLSID"=w668) -> ("error out"=w666:errorcluster)
          }
        }
        n221 = property on="Connect" class="Bool (strict)"(error in=w647, "DisabledEnum"=T3."Enabled" ("Deaktiviert")) -> (error out=w651:errorcluster)  [unwired: 1 in, 1 out]
        n222 = property on="Disconnect" class="Bool (strict)"(error in=w651, "DisabledEnum"=T3."Disabled and Grayed Out" ("Deaktiviert")) -> (error out=w648:errorcluster)  [unwired: 1 in, 1 out]
        n223 = property on="Connected?" class="Bool (strict)"(error in=w648, "Value"=w642) -> (error out=w646:errorcluster)  [unwired: 1 in, 1 out]
        n224 = Release Queue(queue=w654, error in (no error)=w646) -> (error out=w638:errorcluster)  [unwired: 1 in, 2 out]
        n225 = property on="CloseWindow" class="Bool (strict)"(error in=w638) -> (error out=w637:errorcluster, "Value"=w639:bool)  [unwired: 1 in, 1 out]
        n226 = case shown="True" w639 {
          tunnel: w637 -> [w657 w659]
          tunnel: [w657 w658] -> w636
          frame False {
          }
          frame True {
            n227 = Current VI's Path() -> (path=w662:path)
            n228 = Open VI Reference(vi path=w662, error in (no error)=w659) -> (vi reference=w664:refnum<vi>, error out=w663:errorcluster)  [unwired: 4 in]
            n229 = invoke class="VI" method="FP.Close"(reference=w664, error in=w663) -> (reference out=w661:refnum<vi>, error out=w660:errorcluster)  [unwired: 1 in, 1 out]
            n230 = Close Reference(reference=w661, error in (no error)=w660) -> (error out=w658:errorcluster)
          }
        }
      }
    }
    n231 = case shown="\"AllCommands\", Default" w26 {
      selector: w26 -> [_ w43]
      tunnel: w27 -> [_ w44]
      tunnel: w25 -> [w40 w42]
      tunnel: [w40 w41] -> w24
      frame "" {
      }
      frame "AllCommands", Default {
        n232 = Enqueue Element(queue=w44, element=w43, error in (no error)=w42) -> (error out=w41:errorcluster)  [unwired: 1 in, 2 out]
      }
    }
  }
  "error out" <- w5
